vi "Dashboard Main.vi"() -> ()   [LabVIEW 2017]
uses:
  <vilib>/Rock Robotics/WPI/DriverStation/WPI_DriverStationAllianceInfo.ctl
  <vilib>/Rock Robotics/WPI/DriverStation/WPI_DriverStationPositionInfo.ctl
  <vilib>/Rock Robotics/SystemInterfaces/NetworkCommunication/NetComm_MatchType.ctl
  <vilib>/Utility/miscctls.llb/LVRowAndColumnTypeDef.ctl
  <vilib>/event_ctls.llb/eventvkey.ctl
  <vilib>/Rock Robotics/Network Tables/NT Read Numeric Array.vi
  <vilib>/Rock Robotics/Network Tables/NT Write Boolean.vi
  <vilib>/Rock Robotics/WPI/Dashboard/WPI_DashboardLogging Global.vi
panel:
  in  "Camera Name":string(combo)="No Camera Selection"
  out "Camera Info":cluster{"Mbps LED":bool, "Mbps":dbl, "fps":dbl} {"fps" format="%#.1g"; "Mbps" format="%#.1g"}
  in  "Camera Settings":T1={"Frame Rate"=30, "Compression"=30, "Size"=1, "DB Camera Config"=FALSE} {"Frame Rate" scale=1.0..30.0; "Compression" scale=100.0..-1.0; "Size" items=["640x480", "320x240", "160x120"]}
  in  "TCP":refnum<k5>
  out "Robot IP":string
  out "Image Message":string="Timeout in Camera Communications"
  in  "Dashboard Tab":T2(tab)
  out "Cube Lift Height":dbl
  in  "Reset Gyro":bool
  in  "Select Auto":string(combo)="Select Autonomous ..."
  out "NT Connection":bool
  out "MotorChart R":cluster{"Numeric":dbl, "Numeric":dbl}(graph)
  out "MotorChart L":cluster{"Numeric":dbl, "Numeric":dbl}(graph)
  out "MotorSliders R":cluster{"MotorSlide1":dbl, "MotorSlide2":dbl} {"MotorSlide2" scale=-1.0..1.0 scale format="%#_2e"; "MotorSlide1" scale=-1.0..1.0 scale format="%#_2e"}
  out "MotorSliders L":cluster{"MotorSlide1":dbl, "MotorSlide2":dbl} {"MotorSlide2" scale=-1.0..1.0 scale format="%#_2e"; "MotorSlide1" scale=-1.0..1.0 scale format="%#_2e"}
  out "Gyro":dbl(knob) scale=0.0..360.0
  out "JS1 Z":dbl(slide) scale=-1.0..1.0 scale format="%#_2e"
  out "JS1 Graph":cluster{"X":dbl, "Y":dbl}[](graph)
  out "JS1 Buttons":T3
  out "JS2 Z":dbl(slide) scale=-1.0..1.0 scale format="%#_2e"
  out "JS2 Graph":cluster{"X":dbl, "Y":dbl}[](graph)
  out "JS2 Buttons":T3
  out "Mode":T4(ring)=enum."Auto Disabled"
  in  "Rec Mode":enum32{"Stop", "Record", "Playback"}(radio)
  in  "Camera Settings Right":T1={"Frame Rate"=30, "Compression"=30, "Size"=1, "DB Camera Config"=FALSE} {"Frame Rate" scale=1.0..30.0; "Compression" scale=100.0..-1.0; "Size" items=["640x480", "320x240", "160x120"]}
  in  "Camera Name Right":string(combo)="No Camera Selection"
  out "Camera Image Right":T5(plugin-control)
  in  "Cube Lift Up Speed":dbl=10.0 min=0.0 max=10.0 step=1.0
  in  "Robot Lift Speed":dbl=10.0 min=0.0 max=10.0 step=1.0
  in  "H-Wheel Motor Controller Selection":string(combo)="Spark"
  in  "Cube Lift Down Speed":dbl=10.0 min=0.0 max=10.0 step=1.0
  in  "Drive Motor Controller Selection":string(combo)="Talon SRX"
  in  "Y-AXIS":dbl=10.0 min=0.0 max=10.0 step=1.0
  in  "X-AXIS":dbl=10.0 min=0.0 max=10.0 step=1.0
  in  "H-Wheel":dbl=10.0 min=0.0 max=10.0 step=1.0
  out "Event Name":string
  out "Replay Number":u16
  out "Match Type":T6
  out "Match Number":u16
  out "Position":T7
  out "Alliance":T8
  in  "Target Distance":dbl
  out "Inches from Wall":dbl
  in  "Slow Speed":dbl(slide)=0.49999999999999994 scale=0.0..1.0
  in  "Test Slider":dbl(slide) scale=0.0..100.0 scale format="%#_3g"
  in  "On/Off":bool caption="Solenoid"
  in  "Test Name":u16(ring) items=["Select the test to run..."]
  in  "Test Tree":string(tree)
  in  "Motor":cluster{"Value":dbl, "Enable":bool} {"Value" scale=-1.0..1.0 scale format="%#_3g"}
  out "Progress":T9 {"Test Progress" scale=0.0..100.0}
  in  "Rev/Fwd":cluster{"Forward":bool, "Reverse":bool}
  in  "Test Ring":u16(ring) items=["Monochrome", "Color"]
  out "Cmd Status":string
  in  "Execute Command":bool
  in  "Command Params":string[][](table)
  in  "Command Selection":i32(listbox)
  in  "CheckList":i32(listbox)
  out "Tree":string(tree)
  out "Camera Image":T5(plugin-control)
  out "Background":bool
  # "HW"
  # "Joysticks"
  # "Drive Motors"
  # "Front"
  # "Right"
  # "Left"
  # "Back"
  # "HW"
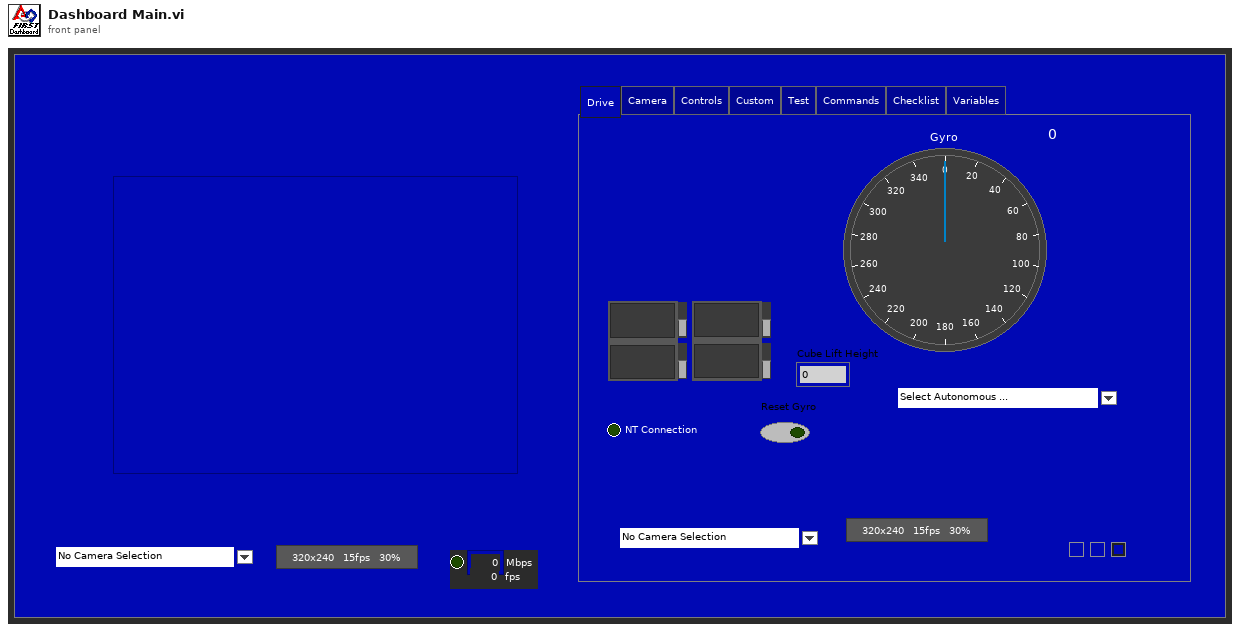
[diagram p1: front panel]
types:
  T1 = cluster{"Frame Rate":i32, "Compression":i32, "Size":u16, "DB Camera Config":bool}
  T2 = enum32{"Drive", "Camera", "Controls", "Custom", "Test", "Commands", "Checklist", "Variables"}
  T3 = cluster{bool, bool, bool, bool, bool, bool, bool, bool, bool, bool, bool, bool}
  T4 = enum8{"Tele-Op Disabled", "Tele-Op Enabled", "Auto Disabled", "Auto Enabled", "Test Disabled", "Test Enabled", "Disconnected", "No Code", "E-Stop"}
  T5 = typedef "IMAQ Image.ctl" = refnum<image>
  T6 = typedef "NetComm_MatchType.ctl" = enum32{"None", "Practice", "Qualification", "Elimination"}
  T7 = typedef "WPI_DriverStationPositionInfo.ctl" = enum16{"1", "2", "3"}
  T8 = typedef "WPI_DriverStationAllianceInfo.ctl" = enum16{"Red", "Blue", "Invalid"}
  T9 = cluster{"Test Progress":u8, "Test Progress Text":string}
  T10 = cluster{"Save Path":path, "Interval (s)":dbl, "Keep":i32}
  T11 = enum32{"Drive", "Camera", "Basic", "Custom", "Test", "Commands", "Checklist", "Variables"}
  T12 = typedef "Image Type" = u32
  T13 = cluster{"IDs":cluster{"RPC field ID":u16, "Unique ID":u16}, "String":string}
  T14 = cluster{"Error Strings":string, "Disable Counts":cluster{u16, u16}, "Rail Faults":cluster{u16, u16, u16}, "Robot IP":string, "DB Mode":u8, "Event Info":cluster{"Name":string, "Type":u8, "Number":u16, "Replay":u8}}
  T15 = cluster{"Storage":cluster{"Disk Free":u64, "RAM Block":u32, "RAM free":u32}, "CPU Utilization":cluster{"CPU % ISR":sgl, "CPU % Time Crit":sgl, "CPU % Timed Str":sgl, "CPU % High":sgl, "CPU % Above":sgl, "CPU % Normal":sgl, "CPU % Low":sgl}, "CAN":cluster{"% Bus Utilization":sgl, "Bus Off Cnt":u32, "TX_FIFO Full Cnt":u32, "Receive Error Cnt":u8, "Transmit Error Cnt":u8}, "HID":cluster{"HID Outputs":u32, "Rumble Low":u16, "Rumble High":u16}[]}
  T16 = cluster{"Status bits":cluster{"Test Mode":bool, "Autonomous":bool, "Enabled":bool, "Code Start":bool, "Brownout":bool, "Reserved 2":bool, "Reserved 3":bool, "E-Stop":bool}, "Code Trace":cluster{"Disabled":bool, "TeleOp":bool, "Auto":bool, "Test":bool}, "Controller Type":enum16{"unknown", "cRIO", "roboRio"}, "Code?":enum16{"unknown", "noCode", "code"}, "Battery V":dbl}
  T17 = cluster{"Control Bits":cluster{"TestMode":bool, "Autonomous":bool, "Enabled":bool, "FMS Present":bool, bool, bool, bool, "E-Stop":bool}, "Team Station ":u8, "Countdown":sgl, "Joystick Values":cluster{"Axes":dbl[], "Buttons":bool[], "POVs":i16[]}[]}
  T18 = cluster{"Axes":dbl[], "Buttons":bool[], "POVs":i16[]}[]
  T19 = cluster{"Axes":dbl[], "Buttons":bool[], "POVs":i16[]}
  T20 = cluster{"Buttons[0]":bool, "Buttons[1]":bool, "Buttons[2]":bool, "Buttons[3]":bool, "Buttons[4]":bool, "Buttons[5]":bool, "Buttons[6]":bool, "Buttons[7]":bool, "Buttons[8]":bool, "Buttons[9]":bool, "Buttons[10]":bool, "Buttons[11]":bool}
  T21 = cluster{"Camera Image":refnum<vi>, "Dashboard Tab":refnum<vi>, "Background":refnum<vi>, "Rec Mode":refnum<vi>, "Test Slider":refnum<vi>, "On/Off ":refnum<vi>, "Test Ring":refnum<vi>, "Rev/Fwd":refnum<vi>, "Test Name":refnum<vi>, "Motor":refnum<vi>, "Progress":refnum<vi>, "CheckList":refnum<vi>, "Tree":refnum<vi>, "Test Tree":refnum<vi>, "Command Params":refnum<vi>, "Command Selection":refnum<vi>, "Execute Command":refnum<vi>, "Cmd Status":refnum<vi>, "Camera Settings":refnum<vi>, "Camera Name":refnum<vi>, "Camera Info":refnum<vi>, "Camera Settings Right":refnum<vi>, "Camera Name Right":refnum<vi>, "Camera Image Right":refnum<vi>}
  T22 = cluster{"Camera Name":string, string, "Saved DB Images Info":cluster{"Save Path":path, "Interval (s)":dbl, "Keep":i32}}
  T23 = cluster{"Camera Name Right":string, string, "Saved DB Images Info":cluster{"Save Path":path, "Interval (s)":dbl, "Keep":i32}}
  T24 = cluster{"Operation":enum16{"Update", "Clear"}, "Color Box":u32}[]
  T25 = typedef "eventvkey.ctl" = enum16{"ASCII", "Enter", "Return", "Shift", "Ctrl", "Alt", "Cmd", "Opt", "Caps", "NumLock", "Clear", "Break", "Up", "Down", "Left", "Right", "Insert", "Delete", "Home", "End", "PageUp", "PageDown", "Escape", "Help", "Pause", "ScrollLock", "F1", "F2", "F3", "F4", "F5", "F6", "F7", "F8", "F9", "F10", "F11", "F12", "F13", "F14", "F15", "F16", "F17", "F18", "F19", "F20", "F21", "F22", "F23", "F24", "Play", "VolumeUp", "VolumeDown", "Mute", "Two Byte Char"}
  T26 = cluster{"Image Size":bool, "Image Type":bool, "Pixel Value":bool, "ROI Information":bool, "Zoom Factor":bool}
  T27 = cluster{"Operation":enum16{"Update", "Clear"}, "Color Box":u32}
  T28 = typedef "LVRowAndColumnTypeDef.ctl" = cluster{"Row":i32, "Column":i32}
  T29 = cluster{"Shift":bool, "Ctrl":bool, "Alt":bool, "Cmd":bool, "Opt":bool}
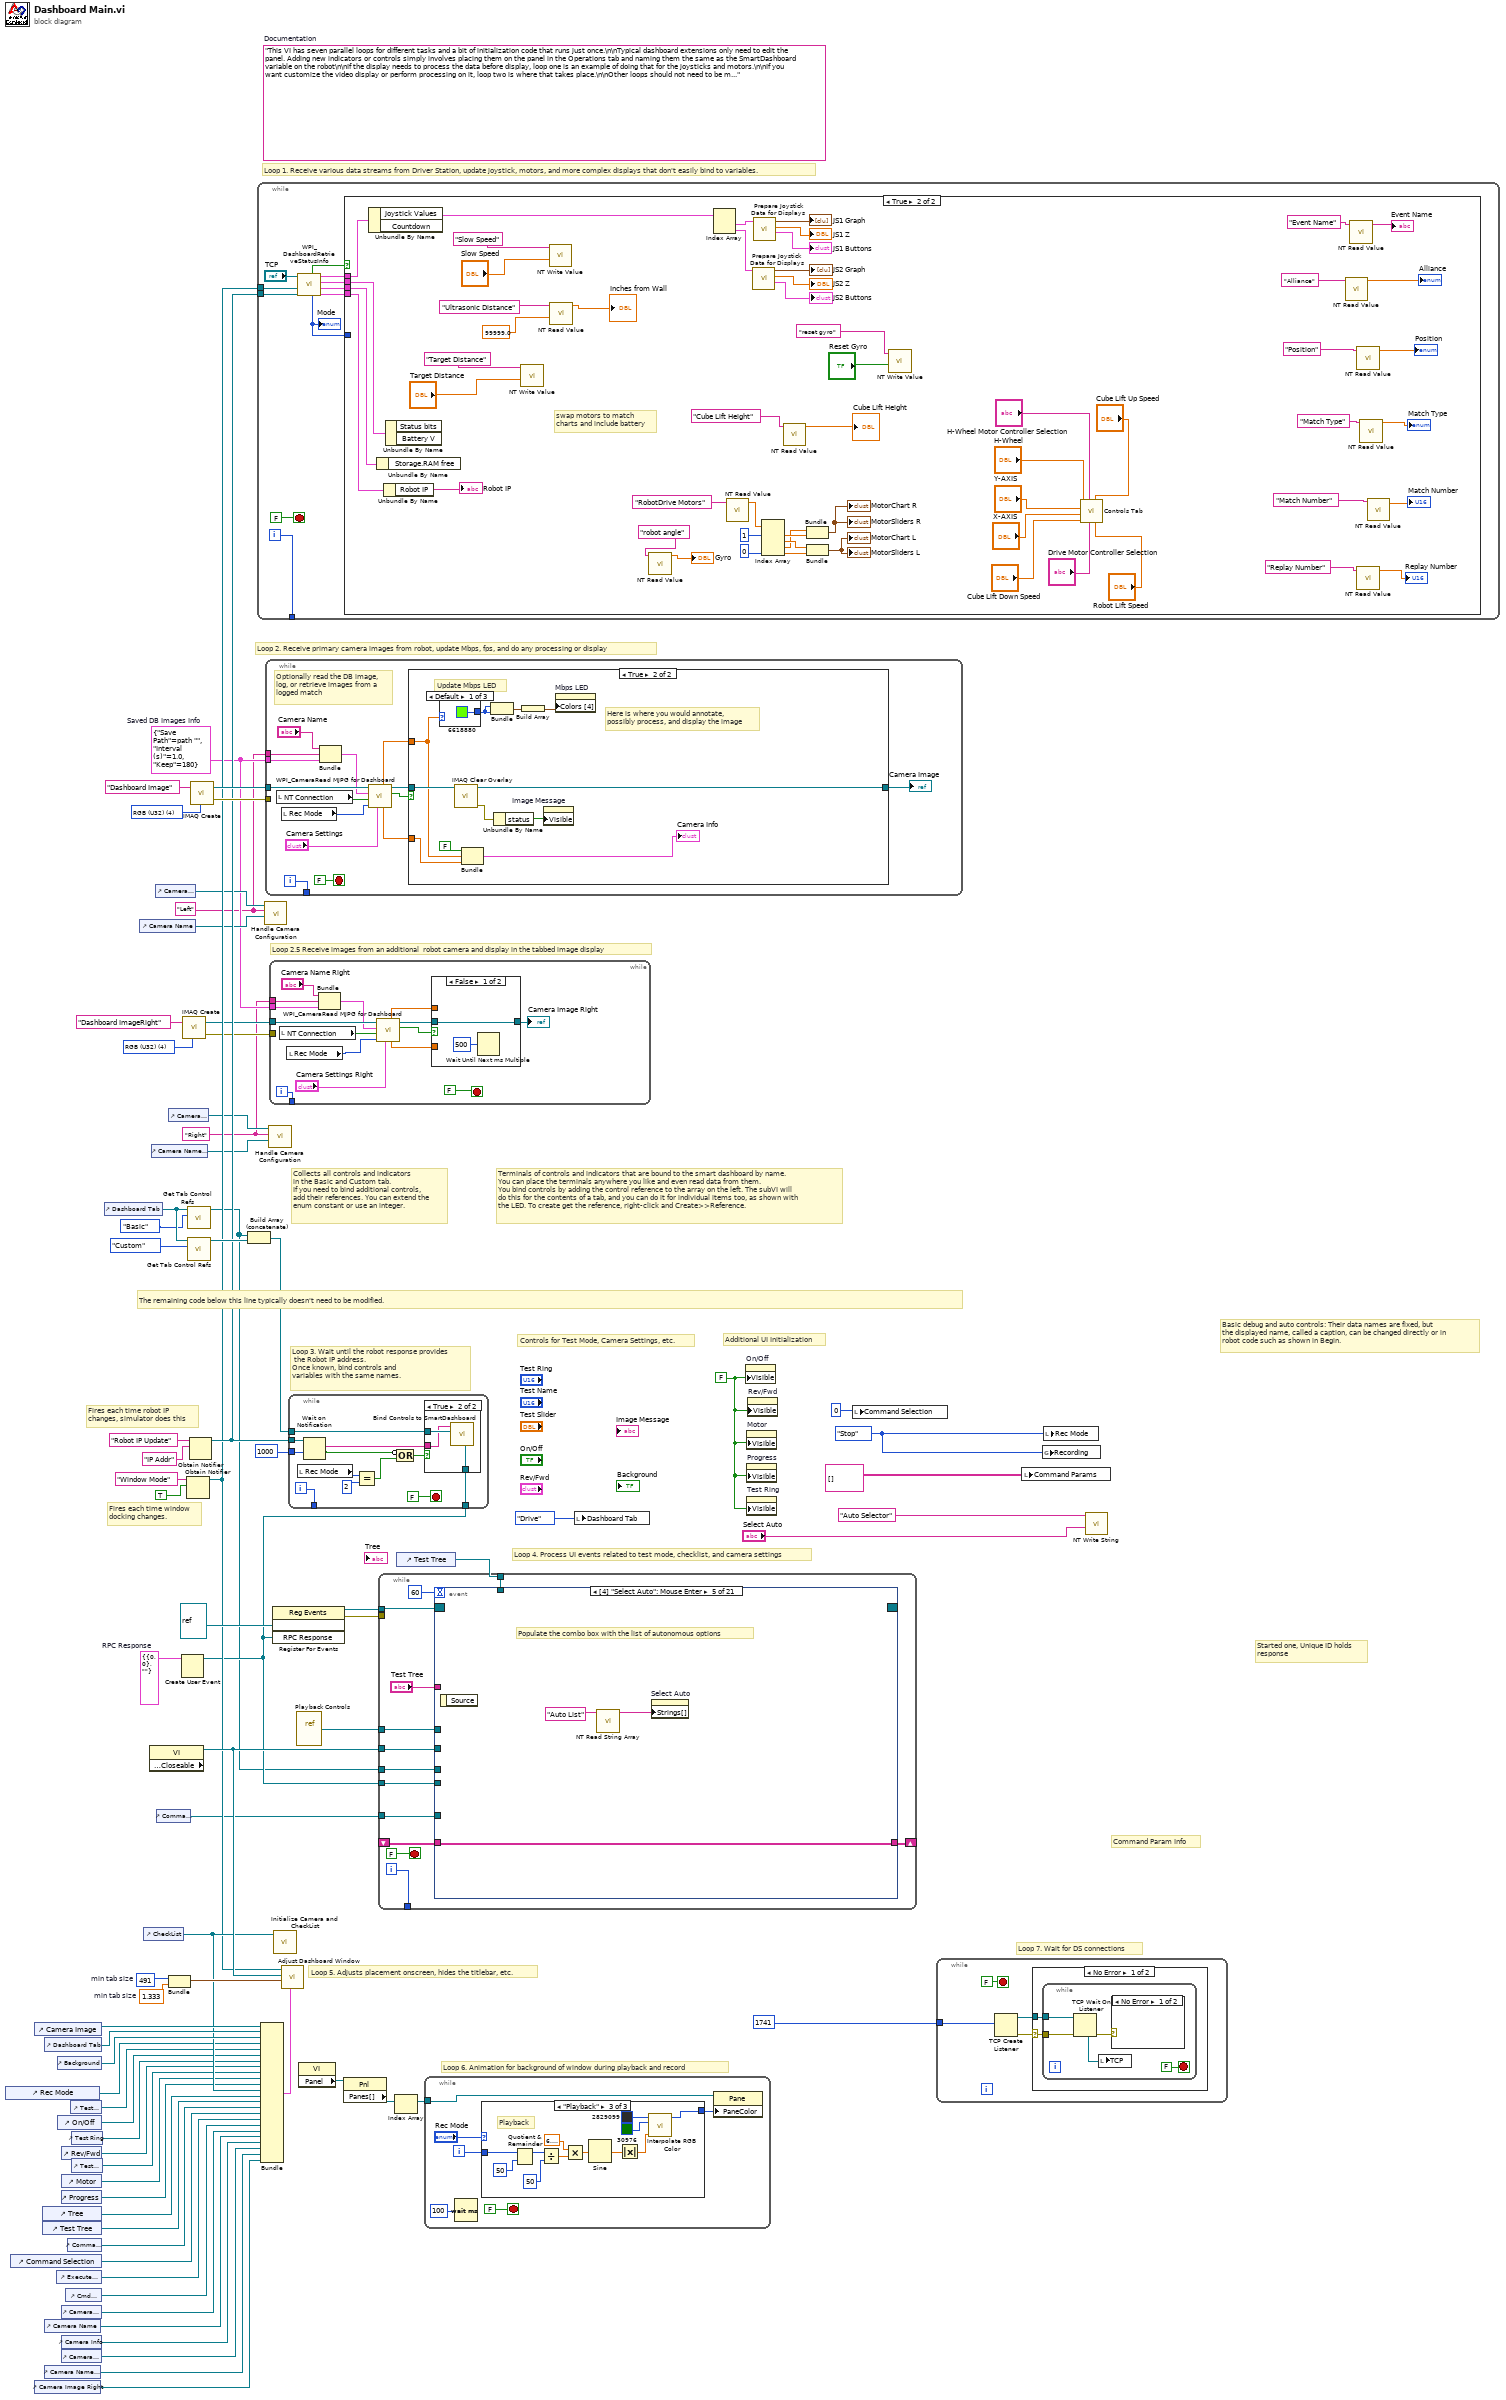
[diagram p0: block diagram]
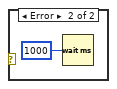
[diagram p3: hidden frame]
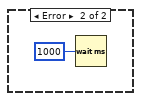
[diagram p4: hidden frame]
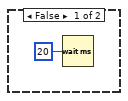
[diagram p5: hidden frame]
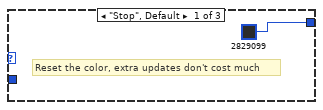
[diagram p6: hidden frame]
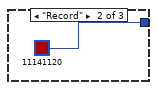
[diagram p7: hidden frame]
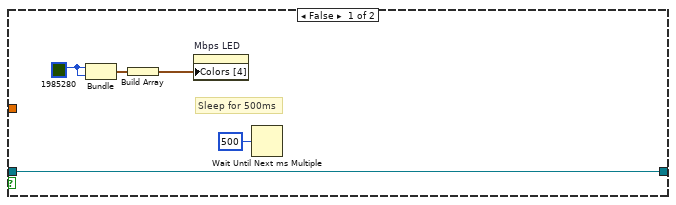
[diagram p9: hidden frame]
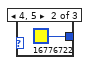
[diagram p10: hidden frame]
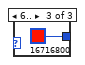
[diagram p11: hidden frame]
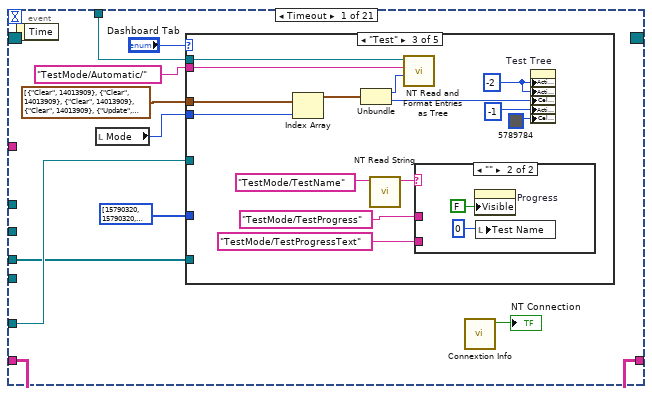
[diagram p12: hidden frame]
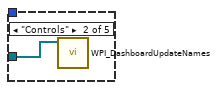
[diagram p14: hidden frame]
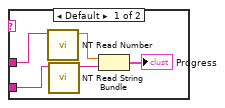
[diagram p15: hidden frame]
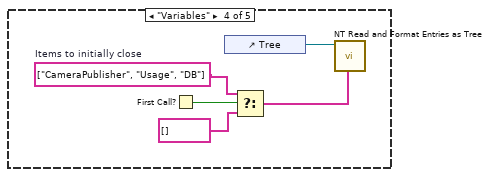
[diagram p16: hidden frame]
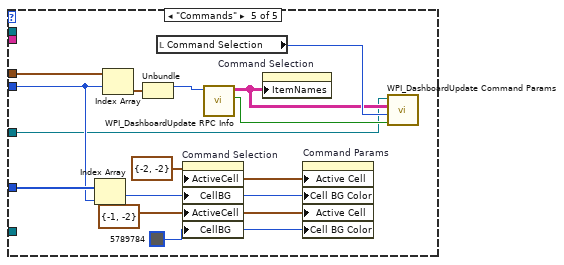
[diagram p17: hidden frame]
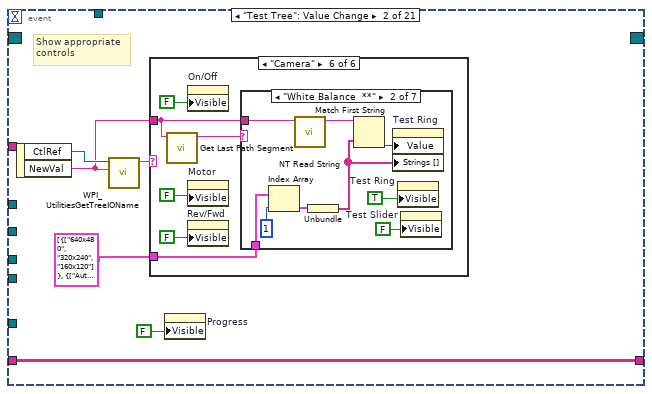
[diagram p18: hidden frame]
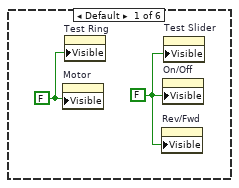
[diagram p19: hidden frame]
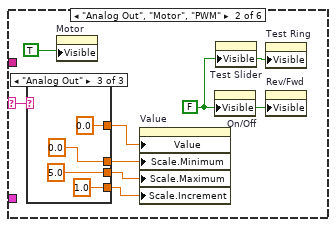
[diagram p20: hidden frame]
diagram:
  w3 = T10 {"Save Path"=path "", "Interval (s)"=1.0, "Keep"=180}  # Saved DB Images Info
  w2 = "Right"
  w1 = "Left"
  w13 = T12 4 items=["Grayscale (U8)", "Grayscale (I16)", "Grayscale (SGL)", "Complex (CSG)", "RGB (U32)", "HSL (U32)", "RGB (U64)"] ("Image Type")
  w29 = T13 {"IDs"={"RPC field ID"=0, "Unique ID"=0}, "String"=""}  # RPC Response
  w52 = 491  # min tab size
  w51 = 1.333  # min tab size
  w59 = enum32{"Stop", "Record", "Playback"}."Stop" ("Rec Mode")
  w36 = FALSE ("Visible")
  (unwired) "This VI has seven parallel loops for different tasks and a bit of initialization code that runs just once.\n\nTypical dashboard extensions only need to edit the panel. Adding new indicators or controls simply involves placing them on the panel in the Operations tab and naming them the same as the SmartDashboard variable on the robot\n\nIf the display needs to process the data before display, loop one is an example of doing that for the joysticks and motors.\n\nIf you want customize the video display or perform processing on it, loop two is where that takes place.\n\nOther loops should not need to be modified. They are pretty standard, and document the task they perform."  # Documentation
  w76 = T12 4 items=["Grayscale (U8)", "Grayscale (I16)", "Grayscale (SGL)", "Complex (CSG)", "RGB (U32)", "HSL (U32)", "RGB (U64)"] ("Image Type")
  # "Loop 2.5 Receive images from an additional  robot camera and display in the tabbed image display"
  # "Command Param Info"
  # "Started one, Unique ID holds\nresponse"
  # "Loop 7. Wait for DS connections"
  # "Basic debug and auto controls: Their data names are fixed, but\nthe displayed name, called a caption, can be changed directly or in\nrobot code such as shown in Begin."
  # "Controls for Test Mode, Camera Settings, etc."
  # "Additional UI Initialization"
  # "Loop 6. Animation for background of window during playback and record"
  # "Fires each time robot IP\nchanges, simulator does this"
  # "Fires each time window\ndocking changes."
  # "Collects all controls and indicators\nin the Basic and Custom tab.\nIf you need to bind additional controls,\nadd their references. You can extend the\nenum constant or use an integer."
  # "The remaining code below this line typically doesn't need to be modified."
  # "Loop 4. Process UI events related to test mode, checklist, and camera settings"
  # "Terminals of controls and indicators that are bound to the smart dashboard by name.\nYou can place the terminals anywhere you like and even read data from them.\nYou bind controls by adding the control reference to the array on the left. The subVI will\ndo this for the contents of a tab, and you can do it for individual items too, as shown with\nthe LED. To create get the reference, right-click and Create>>Reference."
  # "Loop 3. Wait until the robot response provides\n the Robot IP address.\nOnce known, bind controls and\nvariables with the same names."
  # "Loop 5. Adjusts placement onscreen, hides the titlebar, etc."
  # "Loop 1. Receive various data streams from Driver Station, update joystick, motors, and more complex displays that don't easily bind to variables."
  # "Loop 2. Receive primary camera images from robot, update Mbps, fps, and do any processing or display"
  n1 = control-ref of="Rec Mode"() -> (w42:refnum<vi>)
  n2 = control-ref of="Command Selection"() -> (w28:refnum<vi>)
  n3 = control-ref of="Camera Image Right"() -> (w6:refnum<vi>)
  n4 = control-ref of="Camera Image"() -> (w54:refnum<vi>)
  n5 = control-ref of="Tree"() -> (w46:refnum<vi>)
  n6 = control-ref of="Test Tree"() -> (w45:refnum<vi>)
  n7 = control-ref of="Dashboard Tab"() -> (w53:refnum<vi>)
  n8 = control-ref of="Camera Name"() -> (w19:refnum<vi>)
  n9 = control-ref of="Camera Name Right"() -> (w7:refnum<vi>)
  n10 = control-ref of="Execute Command"() -> (w30:refnum<vi>)
  n11 = control-ref of="Background"() -> (w49:refnum<vi>)
  n12 = control-ref of="On/Off"() -> (w40:refnum<vi>)
  n13 = control-ref of="Progress"() -> (w37:refnum<vi>)
  n14 = control-ref of="Camera Settings"() -> (w20:refnum<vi>)
  n15 = control-ref of="Camera Info"() -> (w18:refnum<vi>)
  n16 = control-ref of="Camera Settings Right"() -> (w8:refnum<vi>)
  n17 = control-ref of="Rev/Fwd"() -> (w38:refnum<vi>)
  n18 = control-ref of="Motor"() -> (w43:refnum<vi>)
  n19 = control-ref of="Cmd Status"() -> (w24:refnum<vi>)
  n20 = control-ref of="Command Params"() -> (w31:refnum<vi>)
  n21 = control-ref of="Test Slider"() -> (w41:refnum<vi>)
  n22 = control-ref of="Test Ring"() -> (w39:refnum<vi>)
  n23 = control-ref of="Test Name"() -> (w44:refnum<vi>)
  n24 = control-ref of="Dashboard Tab"() -> (w57:refnum<vi>)
  n25 = control-ref of="Camera Name"() -> (w21:refnum<vi>)
  n26 = control-ref of="CheckList"() -> (w47:refnum<vi>)
  n27 = property class="VI" props=["Front Panel.Closeable"]() -> (reference out=w58:refnum<vi>)  [unwired: 2 in, 2 out]
  n28 = control-ref of="Camera Name Right"() -> (w9:refnum<vi>)
  n29 = control-ref of="Camera Settings"() -> (w22:refnum<vi>)
  n30 = control-ref of="Command Params"() -> (w23:refnum<vi>)
  n31 = control-ref of="Camera Settings Right"() -> (w10:refnum<vi>)
  n32 = Bundle("min tab size"=w52, "min tab size"=w51) -> (w50:cluster{"min tab size":i32, "min tab size":dbl})  [unwired: 1 in]
  n33 = Create User Event(user event datatype=w29) -> (user event=w25:refnum<user-event>)  [unwired: 1 in, 1 out]
  n34 = call "IMAQ Create"("Image Name"="Dashboard ImageRight", "Image Type"=w13) -> ("New Image"=w12:T5, "error out"=w11:errorcluster)  [unwired: 2 in, 1 out]
  n35 = Obtain Notifier(name (unnamed)="Window Mode", notification data type=TRUE) -> (notifier out=w34:refnum<notifier>)  [unwired: 2 in, 2 out]
  n36 = call <vilib>:"Get Tab Control Refs.vi"("Page Index"=T11."Basic" ("Dashboard Tab"), "TabControl in"=w57) -> ("ControlsOnPage"=w17:refnum<vi>[])  [unwired: 9 in]
  n37 = call <vilib>:"Get Tab Control Refs.vi"("Page Index"=T11."Custom" ("Dashboard Tab"), "TabControl in"=w57) -> ("ControlsOnPage"=w56:refnum<vi>[])  [unwired: 9 in]
  n38 = Obtain Notifier(name (unnamed)="Robot IP Update", notification data type="IP Addr" ("name (unnamed)")) -> (notifier out=w35:refnum<notifier>)  [unwired: 2 in, 2 out]
  n39 = call "IMAQ Create"("Image Name"="Dashboard Image", "Image Type"=w76) -> ("New Image"=w74:T5, "error out"=w73:errorcluster)  [unwired: 2 in, 1 out]
  n40 = Build Array (concatenate)(w17, w56) -> (w55:refnum<vi>[])
  n41 = while {
    tunnel: [w86] -> _
    tunnel: w35 -> [w80]
    tunnel: w34 -> [w77]
    i -> [w86]
    stop <- FALSE stop-if-true
    n42 = call <vilib>:"WPI_DashboardRetrieveStatusInfo.vi"("Binding Refnum"=w80, "Window Mode Notifier"=w77, "TCP Cnx"="TCP") -> ("Power and Errors"=w81:T14, "Robot Metrics"=w84:T15, "Status Info"=w85:T16, "Control Info"=w82:T17, "Robot Mode"=w79:T4, "Process?"=w83:bool)  [unwired: 3 in]
    "Mode" <- w79
    n43 = case shown="True" w83 {
      tunnel: w85 -> [_ w145]
      tunnel: w84 -> [_ w144]
      tunnel: w82 -> [_ w143]
      tunnel: w81 -> [_ w142]
      tunnel: w79 -> [_ _]
      frame False {
        n44 = Wait (ms)(milliseconds to wait=u32 20) -> ()  [unwired: 1 out]
      }
      frame True {
        # "swap motors to match\ncharts and include battery"
        n45 = Unbundle By Name(w143) -> ("Joystick Values"=w133:T18)  [unwired: 1 out]
        n46 = Unbundle By Name(w144) -> ()  [unwired: 1 out]
        n47 = Unbundle By Name(w142) -> ("Robot IP"=→"Robot IP":string)
        n48 = Unbundle By Name(w145) -> ()  [unwired: 2 out]
        n49 = call-poly <vilib>:"NT Write Value.vi"("Numeric"="Target Distance", "Name"="Target Distance") -> ()  [unwired: 9 in, 1 out]
        n50 = call-poly <vilib>:"NT Write Value.vi"("Numeric"="Slow Speed", "Name"="Slow Speed") -> ()  [unwired: 9 in, 1 out]
        n51 = call-poly <vilib>:"NT Read Value.vi"("Default Value"=99999.0, "Name"="Ultrasonic Distance") -> ("Numeric"=→"Inches from Wall":dbl)  [unwired: 8 in, 1 out]
        n52 = call-poly <vilib>:"NT Read Value.vi"("Name"="robot angle") -> ("Numeric"=→"Gyro":dbl)  [unwired: 9 in, 1 out]
        n53 = Index Array(array=w133) -> (element #1=w132:T19, element #2=w128:T19)  [unwired: 2 in]
        n54 = call-poly <vilib>:"NT Read Value.vi"("Name"="RobotDrive Motors") -> ("Numeric Array"=w123:dbl[])  [unwired: 9 in, 1 out]
        n55 = call "Prepare Joystick Data for Displays.vi"("Joystick Values"=w128) -> ("Buttons"=→"JS2 Buttons":T20, "Z Axis"=→"JS2 Z":dbl, "Cartesian Data"=→"JS2 Graph":cluster{"X axis":dbl, "X axis":dbl}[])  [unwired: 8 in]
        n56 = call "Prepare Joystick Data for Displays.vi"("Joystick Values"=w132) -> ("Buttons"=→"JS1 Buttons":T20, "Z Axis"=→"JS1 Z":dbl, "Cartesian Data"=→"JS1 Graph":cluster{"X axis":dbl, "X axis":dbl}[])  [unwired: 8 in]
        n57 = Index Array(array=w123, index #1=1, index #4=0) -> (element #1=w137:dbl, element #2=w138:dbl, element #3=w136:dbl, element #4=w141:dbl)  [unwired: 2 in]
        n58 = call-poly <vilib>:"NT Read Value.vi"("Name"="Cube Lift Height") -> ("Numeric"=→"Cube Lift Height":dbl)  [unwired: 9 in, 1 out]
        n59 = Bundle("Numeric"=w136, "Numeric"=w137) -> (→"MotorChart R" →"MotorSliders R":cluster{"Numeric":dbl, "Numeric":dbl})  [unwired: 1 in]
        n60 = Bundle("Numeric"=w138, "Numeric"=w141) -> (→"MotorChart L" →"MotorSliders L":cluster{"Numeric":dbl, "Numeric":dbl})  [unwired: 1 in]
        n61 = call-poly <vilib>:"NT Write Value.vi"("Boolean"="Reset Gyro", "Name"="reset gyro") -> ()  [unwired: 9 in, 1 out]
        n62 = call "Controls Tab.vi"("Robot Lift Motor"="Robot Lift Speed", "Cube Lift Up Motor"="Cube Lift Up Speed", "Motor Controller Selection"="Drive Motor Controller Selection", "H-Wheel Motor Controller Selection"="H-Wheel Motor Controller Selection", "Cube Lift Down Motor"="Cube Lift Down Speed", "X-AXIS"="X-AXIS", "Y-AXIS"="Y-AXIS", "H-Wheel"="H-Wheel") -> ()  [unwired: 4 in]
        n63 = call-poly <vilib>:"NT Read Value.vi"("Name"="Alliance") -> ("Numeric"=→"Alliance":dbl)  [unwired: 9 in, 1 out]
        n64 = call-poly <vilib>:"NT Read Value.vi"("Name"="Event Name") -> ("String"=→"Event Name":string)  [unwired: 9 in, 1 out]
        n65 = call-poly <vilib>:"NT Read Value.vi"("Name"="Position") -> ("Numeric"=→"Position":dbl)  [unwired: 9 in, 1 out]
        n66 = call-poly <vilib>:"NT Read Value.vi"("Name"="Replay Number") -> ("Numeric"=→"Replay Number":dbl)  [unwired: 9 in, 1 out]
        n67 = call-poly <vilib>:"NT Read Value.vi"("Name"="Match Type") -> ("Numeric"=→"Match Type":dbl)  [unwired: 9 in, 1 out]
        n68 = call-poly <vilib>:"NT Read Value.vi"("Name"="Match Number") -> ("Numeric"=→"Match Number":dbl)  [unwired: 9 in, 1 out]
      }
    }
  }
  n69 = Bundle("Camera Image"=w54, "Dashboard Tab"=w53, "Background"=w49, "Rec Mode"=w42, "Test Slider"=w41, "On/Off"=w40, "Test Ring"=w39, "Rev/Fwd"=w38, "Test Name"=w44, "Motor"=w43, "Progress"=w37, "CheckList"=w47, "Tree"=w46, "Test Tree"=w45, "Command Params"=w31, "Command Selection"=w28, "Execute Command"=w30, "Cmd Status"=w24, "Camera Settings"=w20, "Camera Name"=w19, "Camera Info"=w18, "Camera Settings Right"=w8, "Camera Name Right"=w7, "Camera Image Right"=w6) -> (w48:T21)  [unwired: 1 in]
  n70 = call "Handle Camera Configuration.vi"("CameraNameRef"=w21, "Display Name"=w1, "ClusterRef"=w22) -> ()  [unwired: 9 in]
  n71 = while {
    tunnel: w74 -> [w158]
    tunnel: w73 -> [_]
    tunnel: [w159] -> _
    tunnel: w3 -> [w149]
    tunnel: w1 -> [w146]
    i -> [w159]
    stop <- FALSE stop-if-true
    # "Optionally read the DB image,\nlog, or retrieve images from a\nlogged match"
    n72 = local read "NT Connection"() -> (w150:bool)
    n73 = local read "Rec Mode"() -> (w154:enum32{"Stop", "Record", "Playback"})
    n74 = Bundle("Camera Name"="Camera Name", w146, "Saved DB Images Info"=w149) -> (w148:T22)  [unwired: 1 in]
    n75 = call <vilib>:"WPI_CameraRead MJPG for Dashboard.vi"("Camera Settings"="Camera Settings", "Rec Mode"=w154, "NT Connection"=w150, "Capture Info"=w148, "Refnum in"=w158) -> ("Active"=w156:bool, "Refnum out"=w157:T5, "FPS"=w155:dbl, "Bandwidth (Mbps)"=w153:dbl)  [unwired: 3 in]
    n76 = case shown="True" w156 {
      tunnel: w157 -> [w161 w172]
      tunnel: w153 -> [_ w169]
      tunnel: w155 -> [_ w170]
      tunnel: [w161 w166] -> w151
      frame False {
        w163 = u32 1985280 ("Color Box")
        # "Sleep for 500ms"
        n77 = Bundle("Color Box"=w163, "Color Box"=w163) -> (w164:cluster{"Color Box":u32, "Color Box":u32})  [unwired: 1 out]
        n78 = Build Array(w164) -> (w162:cluster{"Color Box":u32, "Color Box":u32}[])
        n79 = property on="Mbps LED" class="Bool (strict)"("Colors [4]"=w162) -> ()  [unwired: 2 in, 2 out]
        n80 = Wait Until Next ms Multiple(millisecond multiple=u32 500) -> ()  [unwired: 1 out]
      }
      frame True {
        # "Here is where you would annotate,\npossibly process, and display the image"
        # "Update Mbps LED"
        n81 = case shown="Default" w169 {
          tunnel: [u32 6618880 ("Color Box") u32 16776722 ("Color Box") u32 16716800 ("Color Box")] -> w173
          frame Default {
          }
          frame 4, 5 {
          }
          frame 6.. {
          }
        }
        n82 = call "IMAQ Clear Overlay"("Image"=w172) -> ("error out"=w175:errorcluster, "Image Out"=w166:T5)  [unwired: 2 in, 7 out]
        n83 = Bundle(FALSE, "Bandwidth (Mbps)"=w169, "FPS"=w170) -> (→"Camera Info":cluster{bool, "Bandwidth (Mbps)":dbl, "FPS":dbl})  [unwired: 1 in]
        n84 = Bundle("Color Box"=w173, "Color Box"=w173) -> (w174:cluster{"Color Box":u32, "Color Box":u32})  [unwired: 1 out]
        n85 = Unbundle By Name(w175) -> ("status"=w176:bool)
        n86 = Build Array(w174) -> (w171:cluster{"Color Box":u32, "Color Box":u32}[])
        n87 = property on="Image Message" class="Str"("Visible"=w176) -> ()  [unwired: 2 in, 2 out]
        n88 = property on="Mbps LED" class="Bool (strict)"("Colors [4]"=w171) -> ()  [unwired: 2 in, 2 out]
      }
    }
    "Camera Image" <- w151
  }
  n89 = call "Handle Camera Configuration.vi"("CameraNameRef"=w9, "Display Name"=w2, "ClusterRef"=w10) -> ()  [unwired: 9 in]
  n90 = while {
    tunnel: w12 -> [w194]
    tunnel: w11 -> [_]
    tunnel: [w189] -> _
    tunnel: w3 -> [w183]
    tunnel: w2 -> [w180]
    i -> [w189]
    stop <- FALSE stop-if-true
    n91 = local read "NT Connection"() -> (w184:bool)
    n92 = local read "Rec Mode"() -> (w193:enum32{"Stop", "Record", "Playback"})
    n93 = Bundle("Camera Name Right"="Camera Name Right", w180, "Saved DB Images Info"=w183) -> (w182:T23)  [unwired: 1 in]
    n94 = call <vilib>:"WPI_CameraRead MJPG for Dashboard.vi"("Camera Settings"="Camera Settings Right", "Rec Mode"=w193, "NT Connection"=w184, "Capture Info"=w182, "Refnum in"=w194) -> ("Active"=w188:bool, "Refnum out"=w191:T5, "FPS"=w186:dbl, "Bandwidth (Mbps)"=w187:dbl)  [unwired: 3 in]
    n95 = case shown="False" w188 {
      tunnel: w191 -> [w195 w197]
      tunnel: w187 -> [_ _]
      tunnel: w186 -> [_ _]
      tunnel: [w195 w197] -> w185
      frame False {
        n96 = Wait Until Next ms Multiple(millisecond multiple=u32 500) -> ()  [unwired: 1 out]
      }
      frame True {
      }
    }
    "Camera Image Right" <- w185
  }
  n97 = register-events(refnum<vi> refnum, w25) -> (reference out=w63:refnum<event-registration>, error out=w62:errorcluster)  [unwired: 2 in]
  n98 = call "Initialize Camera and CheckList.vi"("ListBox in"=w47) -> ()  [unwired: 11 in]
  n99 = call "Adjust Dashboard Window.vi"("Sizing Refnums"=w48, "Size Constraints"=w50, "VI"=w58, "WIn Mode"=w34) -> ()  [unwired: 8 in]
  n100 = while {
    tunnel: w55 -> [w209]
    tunnel: w35 -> [w207]
    tunnel: [w205] -> _
    tunnel: u32 1000 ("milliseconds to wait") -> [w204]
    tunnel: w25 -> [w198]
    i -> [w205]
    stop <- FALSE stop-if-true
    n101 = local read "Rec Mode"() -> (w200:enum32{"Stop", "Record", "Playback"})
    n102 = Wait on Notification(notifier=w207, timeout in ms (-1)=w204) -> (notification=w206:string, timed out?=w202:bool)  [unwired: 2 in, 2 out]
    n103 = Equal?(x=w200, y=u16 2 ("Rec Mode")) -> (x = y?=w201:bool)
    n104 = Compound Arithmetic op=OR(invert w202, w201) -> (w203:bool)
    n105 = case shown="True" w203 {
      tunnel: w209 -> [_ w212]
      tunnel: w206 -> [_ w211]
      tunnel: w198 -> [_ w210]
      frame False {
      }
      frame True {
        n106 = call <vilib>:"Bind Controls to SmartDashboard.vi"("RPC ref"=w210, "Bound Control Refs"=w212, "Server IP Address"=w211) -> ()  [unwired: 9 in]
      }
    }
  }
  n107 = vi-ref "Playback Controls.vi"() -> (w64:refnum<vi>)
  n108 = property class="VI"() -> ("Panel"=w66:refnum<vi>)  [unwired: 2 in, 2 out]
  n109 = property class="Pnl"(reference=w66) -> ("Panes[]"=w67:refnum<vi>[])  [unwired: 1 in, 2 out]
  n110 = Index Array(array=w67) -> (element=w65:refnum<vi>)  [unwired: 1 in]
  n111 = control-ref of="Test Tree"() -> (w68:refnum<vi>)
  n112 = while {
    tunnel: [w222] -> _
    tunnel: w68 -> [w221]
    tunnel: w64 -> [w220]
    tunnel: w63 -> [w219]
    tunnel: w62 -> [_]
    tunnel: w58 -> [w218]
    tunnel: w25 -> [w217]
    tunnel: w23 -> [w216]
    shift-right: [w215] -> _
    shift-left: _ -> [w214]
    tunnel: w17 -> [w213]
    i -> [w222]
    stop <- FALSE stop-if-true
    n113 = event shown="[4] \"Select Auto\": Mouse Enter" {
      selector: w219 -> [_ _ _ _ _ _ _ _ _ _ _ _ _ _ _ _ _ _ _ _ _]
      dyn-events: [_ _ _ _ _ _ _ _ _ _ _ _ _ _ _ _ w482 _ _ _ _] -> _
      timeout: u32 60 ("milliseconds to wait") -> [_ _ _ _ _ _ _ _ _ _ _ _ _ _ _ _ _ _ _ _ _]
      tunnel: w221 -> [w234 _ _ _ _ _ _ _ _ _ _ _ _ _ _ _ _ _ _ _ _]
      tunnel: "Test Tree" -> [_ _ _ _ _ _ _ _ _ _ _ w449 w457 w459 w463 w471 _ _ _ _ _]
      tunnel: w220 -> [_ _ _ _ _ _ _ _ _ _ _ _ _ _ _ _ w484 _ w502 _ _]
      tunnel: w218 -> [_ _ _ _ _ _ _ _ _ _ _ _ _ _ _ _ w480 _ _ _ _]
      tunnel: w217 -> [_ _ _ _ _ _ _ _ _ _ _ _ _ _ _ _ w478 _ _ _ _]
      tunnel: w216 -> [w229 _ _ _ _ _ w400 _ _ _ _ _ _ _ _ _ _ _ _ _ _]
      tunnel: [w228 w277 w379 w384 w393 w397 w398 w407 w417 w424 w436 w448 w455 w458 w462 w470 w477 w497 w499 w503 w516] -> w215
      tunnel: w214 -> [w228 w277 w379 w384 w393 w397 w398 _ _ w424 w436 w448 w455 w458 w462 w470 w477 w497 w499 w503 w516]
      tunnel: w213 -> [w226 _ _ _ _ _ _ _ _ _ _ _ _ _ _ _ _ _ _ _ _]
      event Timeout {
        n114 = event-data() -> ()  [unwired: 1 in, 1 out]
        n115 = local read "Mode"() -> (w231:T4)
        n116 = case shown="\"Test\"" "Dashboard Tab" {
          tunnel: w234 -> [_ _ w250 _ _]
          tunnel: "TestMode/Automatic/" ("Name Pattern") -> [_ _ w249 _ _]
          tunnel: T24 [{"Operation"=enum."Clear", "Color Box"=14013909}, {"Operation"=enum."Clear", "Color Box"=14013909}, {"Operation"=enum."Clear", "Color Box"=14013909}, {"Operation"=enum."Clear", "Color Box"=14013909}, {"Operation"=enum."Update", "Color Box"=14013909}, {"Operation"=enum."Update", "Color Box"=16777215}, {"Operation"=enum."Clear", "Color Box"=14013909}, {"Operation"=enum."Clear", "Color Box"=14013909}, {"Operation"=enum."Clear", "Color Box"=14013909}] -> [_ _ w242 _ w270]
          tunnel: w231 -> [_ _ w241 _ w269]
          tunnel: u32[] [15790320, 15790320, 15790320, 15790320, 16777215, 16777215, 15790320, 15790320, 15790320] -> [_ _ _ _ w275]
          tunnel: w229 -> [_ _ _ _ w263]
          tunnel: w226 -> [_ w236 _ _ _]
          frame "Custom", Default {
          }
          frame "Controls" {
            n117 = call <vilib>:"WPI_DashboardUpdateNames.vi"("Controls on Tab"=w236) -> ()  [unwired: 11 in]
          }
          frame "Test" {
            w248 = -2 ("Active Item:Row Number")
            n118 = Index Array(array=w242, index=w241) -> (element=w243:T27)
            n119 = Unbundle(w243) -> ("Operation"=w244:enum16{"Update", "Clear"}, "Color Box"=w245:u32)
            n120 = call <vilib>:"NT Read String.vi"("Name"="TestMode/TestName") -> ("String"=w239:string)  [unwired: 9 in, 1 out]
            n121 = call <vilib>:"NT Read and Format Entries as Tree.vi"("Operation"=w244, "Name Pattern"=w249, "Tree Refnum"=w250) -> ()  [unwired: 7 in, 2 out]
            n122 = case shown="\"\"" w239 {
              tunnel: "TestMode/TestProgress" ("Name") -> [w252 _]
              tunnel: "TestMode/TestProgressText" ("Name") -> [w251 _]
              frame Default {
                n123 = call <vilib>:"NT Read Number.vi"("Name"=w252) -> ("Numeric"=w253:dbl)  [unwired: 9 in, 1 out]
                n124 = call <vilib>:"NT Read String.vi"("Name"=w251) -> ("String"=w254:string)  [unwired: 9 in, 1 out]
                n125 = Bundle("Numeric"=w253, "String"=w254) -> (→"Progress":cluster{"Numeric":dbl, "String":string})  [unwired: 1 in]
              }
              frame "" {
                n126 = property on="Progress" class="Clust (strict)"("Visible"=FALSE) -> ()  [unwired: 2 in, 2 out]
                n127 = local write "Test Name"(u16 0) -> ()
              }
            }
            n128 = property on="Test Tree" class="Tree (strict)"("Active Item Row Number"=w248, "ActiveColNum"=w248, "CellBG"=w245, "Active Item Row Number"=-1 ("Active Item:Row Number"), "CellBG"=u32 5789784 ("Color Box")) -> ()  [unwired: 2 in, 2 out]
          }
          frame "Variables" {
            w260 = string[] ["CameraPublisher", "Usage", "DB"]  # Items to initially close
            n129 = First Call?() -> (First Call?: T/F=w261:bool)
            n130 = control-ref of="Tree"() -> (w262:refnum<vi>)
            n131 = Select(t=w260, s=w261, f=string[] []) -> (s? t:f=w258:string[])
            n132 = call <vilib>:"NT Read and Format Entries as Tree.vi"("Tags to  Close"=w258, "Tree Refnum"=w262) -> ()  [unwired: 8 in, 2 out]
          }
          frame "Commands" {
            w271 = u32 5789784 ("Color Box")
            w272 = T28 {"Row"=-1, "Column"=-2} ("Active Cell:Active Cell")
            w274 = T28 {"Row"=-2, "Column"=-2} ("Active Cell:Active Cell")
            n133 = Index Array(array=w275, index=w269) -> (element=w273:u32)
            n134 = Index Array(array=w270, index=w269) -> (element=w268:T27)
            n135 = Unbundle(w268) -> ("Operation"=w267:enum16{"Update", "Clear"})  [unwired: 1 out]
            n136 = local read "Command Selection"() -> (w266:i32)
            n137 = property on="Command Selection" class="MCListbox (strict)"("ActiveCell"=w274, "CellBG"=w273, "ActiveCell"=w272, "CellBG"=w271) -> ()  [unwired: 2 in, 2 out]
            n138 = call <vilib>:"WPI_DashboardUpdate RPC Info.vi"("Operation"=w267) -> ("update"=w265:bool, "commands"=w264:string[][])  [unwired: 9 in]
            n139 = property on="Command Selection" class="MCListbox (strict)"("ItemNames"=w264) -> ()  [unwired: 2 in, 2 out]
            n140 = property on="Command Params" class="Tbl (strict)"("Active Cell"=w274, "Cell BG Color"=w273, "Active Cell"=w272, "Cell BG Color"=w271) -> ()  [unwired: 2 in, 2 out]
            n141 = call <vilib>:"WPI_DashboardUpdate Command Params.vi"("Update"=w265, "NewVal"=w266, "Commands"=w264, "Param Tbl"=w263) -> ()  [unwired: 7 in, 1 out]
          }
        }
        n142 = call <vilib>:"Connextion Info.vi"() -> ("Connected"=→"NT Connection":bool)  [unwired: 10 in, 1 out]
      }
      event "Test Tree": Value Change {
        # "Show appropriate\ncontrols"
        n143 = event-data() -> ("CtlRef"=w280:refnum<vi>, "NewVal"=w278:string)  [unwired: 1 in]
        n144 = call <vilib>:"WPI_UtilitiesGetTreeIOName.vi"("NewVal"=w278, "TreeControl in"=w280) -> ("I/O Name"=w281:string)  [unwired: 9 in]
        n145 = case shown="\"Camera\"" w281 {
          selector: w281 -> [_ w288 _ w310 w319 _]
          tunnel: w278 -> [_ _ w307 w309 _ w326]
          tunnel: cluster{string[]}[] [{["640x480", "320x240", "160x120"]}, {["Auto", "Fixed indoor", "Fixed outdoor 1", "Fixed outdoor 2", "Fixed fluorescent 1", "Fixed fluorescent 2", "Hold current"]}, {["Auto", "Flicker-free 50 Hz", "Flicker-free 60 Hz", "Hold current"]}, {["None", "Prioritize frame rate", "Prioritize image quality"]}, {["Monochrome", "Color"]}] -> [_ _ _ _ _ w325]
          frame Default {
            w283 = FALSE ("Visible")
            w282 = FALSE ("Visible")
            n146 = property on="Motor" class="Clust (strict)"("Visible"=w282) -> ()  [unwired: 2 in, 2 out]
            n147 = property on="Test Ring" class="Ring (strict)"("Visible"=w282) -> ()  [unwired: 2 in, 2 out]
            n148 = property on="Rev/Fwd" class="Clust (strict)"("Visible"=w283) -> ()  [unwired: 2 in, 2 out]
            n149 = property on="On/Off" class="Bool (strict)"("Visible"=w283) -> ()  [unwired: 2 in, 2 out]
            n150 = property on="Test Slider" class="Slide (strict)"("Visible"=w283) -> ()  [unwired: 2 in, 2 out]
          }
          frame "Analog Out", "Motor", "PWM" {
            w289 = FALSE ("Visible")
            n151 = case shown="\"Analog Out\"" w288 {
              tunnel: [1.0 ("Value") -1.0 ("Value") 0.0 ("Value")] -> w287
              tunnel: [255.0 ("Value") 1.0 ("Value") 5.0 ("Value")] -> w286
              tunnel: [128.0 ("Value") 0.0 ("Value") 0.0 ("Value")] -> w285
              tunnel: [64.0 ("Value") 0.5 ("Value") 1.0 ("Value")] -> w284
              frame "PWM" {
              }
              frame "Motor", Default {
              }
              frame "Analog Out" {
              }
            }
            n152 = property on="Motor" class="Clust (strict)"("Visible"=TRUE) -> ()  [unwired: 2 in, 2 out]
            n153 = property on="Value" class="Slide (strict)"("Value"=w285, "Scale.Minimum"=w287, "Scale.Maximum"=w286, "Scale.Increment"=w284) -> ()  [unwired: 2 in, 2 out]
            n154 = property on="On/Off" class="Bool (strict)"("Visible"=w289) -> ()  [unwired: 2 in, 2 out]
            n155 = property on="Test Slider" class="Slide (strict)"("Visible"=w289) -> ()  [unwired: 2 in, 2 out]
            n156 = property on="Test Ring" class="Ring (strict)"("Visible"=w289) -> ()  [unwired: 2 in, 2 out]
            n157 = property on="Rev/Fwd" class="Clust (strict)"("Visible"=w289) -> ()  [unwired: 2 in, 2 out]
          }
          frame "Servo" {
            w305 = FALSE ("Visible")
            n158 = call <vilib>:"NT Read Number.vi"("Name"=w307) -> ("Numeric"=w306:dbl)  [unwired: 9 in, 1 out]
            n159 = property on="Test Slider" class="Slide (strict)"("Visible"=TRUE, "Scale.Maximum"=170.0 ("Scale.Range:Maximum")) -> ()  [unwired: 2 in, 2 out]
            n160 = local write "Test Slider"(w306) -> ()
            n161 = property on="Motor" class="Clust (strict)"("Visible"=w305) -> ()  [unwired: 2 in, 2 out]
            n162 = property on="Rev/Fwd" class="Clust (strict)"("Visible"=w305) -> ()  [unwired: 2 in, 2 out]
            n163 = property on="On/Off" class="Bool (strict)"("Visible"=w305) -> ()  [unwired: 2 in, 2 out]
            n164 = property on="Test Ring" class="Ring (strict)"("Visible"=w305) -> ()  [unwired: 2 in, 2 out]
          }
          frame "Relay", "Solenoid" {
            w308 = FALSE ("Visible")
            n165 = property on="Motor" class="Clust (strict)"("Visible"=w308) -> ()  [unwired: 2 in, 2 out]
            n166 = property on="Test Slider" class="Slide (strict)"("Visible"=w308) -> ()  [unwired: 2 in, 2 out]
            n167 = Search and Replace String(input string=w309, search string="/Value  **", replace string="/Direction") -> (result string=w315:string)  [unwired: 5 in, 3 out]
            n168 = property on="Test Ring" class="Ring (strict)"("Visible"=w308) -> ()  [unwired: 2 in, 2 out]
            n169 = call <vilib>:"NT Read String.vi"("Name"=w315) -> ("String"=w313:string)  [unwired: 9 in, 1 out]
            n170 = Equal?(x="Both directions", y=w313) -> (x = y?=w311:bool)
            n171 = Not(x=w311) -> (.not. x?=w312:bool)
            n172 = property on="Rev/Fwd" class="Clust (strict)"("Visible"=w311) -> ()  [unwired: 2 in, 2 out]
            n173 = property on="On/Off" class="Bool (strict)"("Visible"=w312, "Caption.Text"=w310) -> ()  [unwired: 2 in, 2 out]
          }
          frame "Compressor", "Digital Out" {
            w318 = FALSE ("Visible")
            # "Get direction and finish"
            n174 = property on="Motor" class="Clust (strict)"("Visible"=w318) -> ()  [unwired: 2 in, 2 out]
            n175 = property on="Test Slider" class="Slide (strict)"("Visible"=w318) -> ()  [unwired: 2 in, 2 out]
            n176 = property on="Test Ring" class="Ring (strict)"("Visible"=w318) -> ()  [unwired: 2 in, 2 out]
            n177 = property on="On/Off" class="Bool (strict)"("Visible"=TRUE, "Caption.Text"=w319) -> ()  [unwired: 2 in, 2 out]
            n178 = property on="Rev/Fwd" class="Clust (strict)"("Visible"=FALSE) -> ()  [unwired: 2 in, 2 out]
          }
          frame "Camera" {
            n179 = call <vilib>:"Get Last Path Segment.vi"("String in"=w326) -> ("String out"=w327:string)  [unwired: 10 in]
            n180 = property on="On/Off" class="Bool (strict)"("Visible"=FALSE) -> ()  [unwired: 2 in, 2 out]
            n181 = property on="Motor" class="Clust (strict)"("Visible"=FALSE) -> ()  [unwired: 2 in, 2 out]
            n182 = property on="Rev/Fwd" class="Clust (strict)"("Visible"=FALSE) -> ()  [unwired: 2 in, 2 out]
            n183 = case shown="\"White Balance  **\"" w327 {
              tunnel: w326 -> [w333 w342 w351 w360 w369 _ w375]
              tunnel: w325 -> [w331 w339 w348 w357 w366 _ _]
              frame "Size  **" {
                n184 = Index Array(array=w331) -> (element=w330:cluster{string[]})  [unwired: 1 in]
                n185 = call <vilib>:"NT Read String.vi"("Name"=w333) -> ("String"=w332:string)  [unwired: 9 in, 1 out]
                n186 = Unbundle(w330) -> (w328:string[])
                n187 = Match First String(2:w328, 3:w332) -> (0:w329:i32)  [unwired: 1 out]
                n188 = property on="Test Ring" class="Ring (strict)"("Value"=w329, "Strings []"=w328) -> ()  [unwired: 2 in, 2 out]
                n189 = property on="Test Ring" class="Ring (strict)"("Visible"=TRUE) -> ()  [unwired: 2 in, 2 out]
                n190 = property on="Test Slider" class="Slide (strict)"("Visible"=FALSE) -> ()  [unwired: 2 in, 2 out]
              }
              frame "White Balance  **" {
                n191 = Index Array(array=w339, index=1) -> (element=w340:cluster{string[]})
                n192 = call <vilib>:"NT Read String.vi"("Name"=w342) -> ("String"=w341:string)  [unwired: 9 in, 1 out]
                n193 = Unbundle(w340) -> (w337:string[])
                n194 = Match First String(2:w337, 3:w341) -> (0:w336:i32)  [unwired: 1 out]
                n195 = property on="Test Ring" class="Ring (strict)"("Value"=w336, "Strings []"=w337) -> ()  [unwired: 2 in, 2 out]
                n196 = property on="Test Ring" class="Ring (strict)"("Visible"=TRUE) -> ()  [unwired: 2 in, 2 out]
                n197 = property on="Test Slider" class="Slide (strict)"("Visible"=FALSE) -> ()  [unwired: 2 in, 2 out]
              }
              frame "Exposure  **" {
                n198 = Index Array(array=w348, index=2) -> (element=w349:cluster{string[]})
                n199 = call <vilib>:"NT Read String.vi"("Name"=w351) -> ("String"=w350:string)  [unwired: 9 in, 1 out]
                n200 = Unbundle(w349) -> (w345:string[])
                n201 = Match First String(2:w345, 3:w350) -> (0:w346:i32)  [unwired: 1 out]
                n202 = property on="Test Ring" class="Ring (strict)"("Value"=w346, "Strings []"=w345) -> ()  [unwired: 2 in, 2 out]
                n203 = property on="Test Ring" class="Ring (strict)"("Visible"=TRUE) -> ()  [unwired: 2 in, 2 out]
                n204 = property on="Test Slider" class="Slide (strict)"("Visible"=FALSE) -> ()  [unwired: 2 in, 2 out]
              }
              frame "Exposure Priority  **" {
                n205 = Index Array(array=w357, index=3) -> (element=w358:cluster{string[]})
                n206 = call <vilib>:"NT Read String.vi"("Name"=w360) -> ("String"=w359:string)  [unwired: 9 in, 1 out]
                n207 = Unbundle(w358) -> (w354:string[])
                n208 = Match First String(2:w354, 3:w359) -> (0:w355:i32)  [unwired: 1 out]
                n209 = property on="Test Ring" class="Ring (strict)"("Value"=w355, "Strings []"=w354) -> ()  [unwired: 2 in, 2 out]
                n210 = property on="Test Ring" class="Ring (strict)"("Visible"=TRUE) -> ()  [unwired: 2 in, 2 out]
                n211 = property on="Test Slider" class="Slide (strict)"("Visible"=FALSE) -> ()  [unwired: 2 in, 2 out]
              }
              frame "Color Enable  **" {
                n212 = Index Array(array=w366, index=4) -> (element=w367:cluster{string[]})
                n213 = call <vilib>:"NT Read String.vi"("Name"=w369) -> ("String"=w368:string)  [unwired: 9 in, 1 out]
                n214 = Unbundle(w367) -> (w363:string[])
                n215 = Match First String(2:w363, 3:w368) -> (0:w364:i32)  [unwired: 1 out]
                n216 = property on="Test Ring" class="Ring (strict)"("Value"=w364, "Strings []"=w363) -> ()  [unwired: 2 in, 2 out]
                n217 = property on="Test Ring" class="Ring (strict)"("Visible"=TRUE) -> ()  [unwired: 2 in, 2 out]
                n218 = property on="Test Slider" class="Slide (strict)"("Visible"=FALSE) -> ()  [unwired: 2 in, 2 out]
              }
              frame Default {
                n219 = property on="Test Ring" class="Ring (strict)"("Visible"=FALSE) -> ()  [unwired: 2 in, 2 out]
                n220 = property on="Test Slider" class="Slide (strict)"("Visible"=FALSE) -> ()  [unwired: 2 in, 2 out]
              }
              frame "Brightness  **", "Color Level  **", "Compression  **", "FPS  **", "Sharpness  **" {
                n221 = call <vilib>:"NT Read Number.vi"("Name"=w375) -> ("Numeric"=w374:dbl)  [unwired: 9 in, 1 out]
                n222 = local write "Test Slider"(w374) -> ()
                n223 = property on="Test Slider" class="Slide (strict)"("Visible"=TRUE, "Scale.Maximum"=100.0 ("Scale.Range:Maximum")) -> ()  [unwired: 2 in, 2 out]
                n224 = property on="Test Ring" class="Ring (strict)"("Visible"=FALSE) -> ()  [unwired: 2 in, 2 out]
              }
            }
          }
        }
        n225 = property on="Progress" class="Clust (strict)"("Visible"=FALSE) -> ()  [unwired: 2 in, 2 out]
      }
      event "Test Name": Mouse Enter {
        # "Populate the ring with the list of tests"
        n226 = event-data() -> ()  [unwired: 1 in, 1 out]
        n227 = call <vilib>:"NT Read String Array.vi"("Name"="TestMode/TestList") -> ("String Array"=w383:string[])  [unwired: 9 in, 1 out]
        n228 = Build Array (concatenate)("Select the test to run...", w383) -> (w382:string[])
        n229 = property on="Test Name" class="Ring (strict)"("Strings []"=w382) -> ()  [unwired: 2 in, 2 out]
      }
      event "Test Name": Value Change {
        w385 = FALSE ("Visible")
        # "Tell the robot the test name to run"
        n230 = event-data() -> ("NewVal"=w389:u16)  [unwired: 1 in]
        n231 = property on="Test Name" class="Ring (strict)"() -> ("Strings []"=w390:string[])  [unwired: 2 in, 2 out]
        n232 = local write "Progress"(T9 {"Test Progress"=0, "Test Progress Text"=""} ("Progress")) -> ()
        n233 = Index Array(array=w390, index=w389) -> (element=w388:string)
        n234 = call <vilib>:"NT Write String.vi"("String"=w388, "Name"="TestMode/TestName") -> ()  [unwired: 9 in, 1 out]
        n235 = property on="Progress" class="Clust (strict)"("Visible"=TRUE) -> ()  [unwired: 2 in, 2 out]
        n236 = property on="Motor" class="Clust (strict)"("Visible"=w385) -> ()  [unwired: 2 in, 2 out]
        n237 = property on="Test Slider" class="Slide (strict)"("Visible"=w385) -> ()  [unwired: 2 in, 2 out]
        n238 = property on="On/Off" class="Bool (strict)"("Visible"=w385) -> ()  [unwired: 2 in, 2 out]
        n239 = property on="Rev/Fwd" class="Clust (strict)"("Visible"=w385) -> ()  [unwired: 2 in, 2 out]
        n240 = property on="Test Ring" class="Ring (strict)"("Visible"=w385) -> ()  [unwired: 2 in, 2 out]
      }
      event "Select Auto": Mouse Enter {
        # "Populate the combo box with the list of autonomous options"
        n241 = event-data() -> ()  [unwired: 1 in, 1 out]
        n242 = call <vilib>:"NT Read String Array.vi"("Name"="Auto List") -> ("String Array"=w392:string[])  [unwired: 9 in, 1 out]
        n243 = property on="Select Auto" class="CmbBox"("Strings[]"=w392) -> ()  [unwired: 2 in, 2 out]
      }
      event "Select Auto": Value Change {
        # "User modified the Auto Selection. Write to NT variable so robot knows."
        n244 = event-data() -> ("NewVal"=w395:string)  [unwired: 1 in]
        n245 = call <vilib>:"NT Write String.vi"("String"=w395, "Name"="Auto Selector") -> ()  [unwired: 9 in, 1 out]
      }
      event "Command Selection": Value Change {
        # "Get the params and show in table"
        n246 = event-data() -> ("NewVal"=w401:i32)  [unwired: 1 in]
        n247 = property on="Command Selection" class="MCListbox (strict)"() -> ("ItemNames"=w399:string[][])  [unwired: 2 in, 2 out]
        n248 = call <vilib>:"WPI_DashboardUpdate Command Params.vi"("NewVal"=w401, "Commands"=w399, "Param Tbl"=w400) -> ()  [unwired: 8 in, 1 out]
      }
      event "Execute Command": Value Change {
        # "Started one, Unique ID holds\nresponse"
        n249 = event-data() -> ()  [unwired: 1 in, 1 out]
        n250 = property on="Command Selection" class="MCListbox (strict)"() -> ("ItemNames"=w412:string[][])  [unwired: 2 in, 2 out]
        n251 = Index Array(array=w412, index (row)="Command Selection", index (col)=0) -> (element=w410:string)
        n252 = call <vilib>:"Invoke Commands.vi"("Command Params"="Command Params", "Function Name"=w410) -> ("Params"=w406:u8, "Started"=w405:bool)  [unwired: 7 in, 1 out]
        n253 = Array Subset(array="Command Params", length (row)=w406) -> (w407:string[][])  [unwired: 3 in]
        n254 = Select(t="Executing" ("Cmd Status"), s=w405, f="" ("Cmd Status")) -> (s? t:f=→"Cmd Status":string)
      }
      event "Command Selection": Double Click {
        n255 = event-data() -> ("Row"=w420:i32)  [unwired: 1 in]
        n256 = property on="Command Selection" class="MCListbox (strict)"() -> ("ItemNames"=w423:string[][])  [unwired: 2 in, 2 out]
        n257 = local read "Command Params"() -> (w419:string[][])
        n258 = Index Array(array=w423, index (row)=w420, index (col)=0) -> (element=w421:string)
        n259 = call <vilib>:"Invoke Commands.vi"("Command Params"=w419, "Function Name"=w421) -> ("Params"=w418:u8, "Started"=w413:bool)  [unwired: 7 in, 1 out]
        n260 = Array Subset(array=w419, length (row)=w418) -> (w417:string[][])  [unwired: 3 in]
        n261 = Select(t="Executing" ("Cmd Status"), s=w413, f="" ("Cmd Status")) -> (s? t:f=w414:string)
        n262 = local write "Cmd Status"(w414) -> ()
      }
      event "CheckList": Double Click {
        # "Shift clears all"
        # "Update symbols on the listbox"
        n263 = event-data() -> ("PlatMods.Shift"=w425:bool, "Row"=w427:i32)  [unwired: 1 in]
        n264 = case shown="True" w425 {
          tunnel: w427 -> [w431 _]
          tunnel: 1 -> [w430 _]
          frame False {
            n265 = property on="CheckList" class="LstBox (strict)"() -> ("Item Symbols"=w429:i32[])  [unwired: 2 in, 2 out]
            n266 = Replace Array Subset(array=w429, new element=w430, index=w431) -> (w428:i32[])
            n267 = property on="CheckList" class="LstBox (strict)"("Item Symbols"=w428) -> ()  [unwired: 2 in, 2 out]
          }
          frame True {
            w432 = 0 ("Top Row")
            n268 = property on="CheckList" class="LstBox (strict)"() -> ("Number of Rows"=w434:u32)  [unwired: 2 in, 2 out]
            n269 = Initialize Array(0, w434) -> (w433:i32[])
            n270 = property on="CheckList" class="LstBox (strict)"("Top Row"=w432, "Value"=w432, "Item Symbols"=w433) -> ()  [unwired: 2 in, 2 out]
          }
        }
      }
      event "CheckList": Key Down {
        # "Update symbols on the listbox\nLeft and right keys check and uncheck"
        n271 = event-data() -> ("VKey"=w438:T25)  [unwired: 1 in]
        n272 = case shown="\"Left\", \"Right\"" w438 {
          selector: w438 -> [w443 _]
          tunnel: eventvkey."Left" ("VKey") -> [w441 _]
          frame "Left", "Right" {
            n273 = Equal?(x=w441, y=w443) -> (x = y?=w442:bool)
            n274 = Select(t=0, s=w442, f=1) -> (s? t:f=w444:i32)
            n275 = property on="CheckList" class="LstBox (strict)"() -> ("Item Symbols"=w447:i32[])  [unwired: 2 in, 2 out]
            n276 = Replace Array Subset(array=w447, new element=w444, index="CheckList") -> (w446:i32[])
            n277 = property on="CheckList" class="LstBox (strict)"("Item Symbols"=w446) -> ()  [unwired: 2 in, 2 out]
          }
          frame Default {
          }
        }
      }
      event "Motor.Enable": Value Change {
        # "When the test mode otor enable helper is set, update that\ntree row item's value"
        n278 = event-data() -> ("NewVal"=w453:bool)  [unwired: 1 in]
        n279 = Unbundle("Motor") -> ("Value"=w452:dbl)  [unwired: 1 out]
        n280 = Select(t=w452, s=w453, f=0.0) -> (s? t:f=w450:dbl)
        n281 = call <vilib>:"NT Write Number.vi"("Numeric"=w450, "Name"=w449) -> ()  [unwired: 9 in, 1 out]
      }
      event "Test Slider": Value Change {
        # "When the test mode slider helper is set, update that\ntree row item's value"
        n282 = event-data() -> ("NewVal"=w456:dbl)  [unwired: 1 in]
        n283 = call <vilib>:"NT Write Number.vi"("Numeric"=w456, "Name"=w457) -> ()  [unwired: 9 in, 1 out]
      }
      event "On/Off": Value Change {
        # "When the test mode on/off helper value is set, update that\ntree row item's value"
        n284 = event-data() -> ("NewVal"=w461:bool)  [unwired: 1 in]
        n285 = Boolean To (0,1)(Boolean=w461) -> (0, 1=w460:i16)
        n286 = call <vilib>:"NT Write Number.vi"("Numeric"=w460, "Name"=w459) -> ()  [unwired: 9 in, 1 out]
      }
      event "Rev/Fwd": Value Change {
        # "When the test mode helper value for relays is set, update that\ntree row item's value"
        n287 = event-data() -> ("NewVal.Forward"=w469:bool, "NewVal.Reverse"=w468:bool)  [unwired: 1 in]
        n288 = Boolean To (0,1)(Boolean=w469) -> (0, 1=w465:i16)
        n289 = Boolean To (0,1)(Boolean=w468) -> (0, 1=w467:i16)
        n290 = Negate(x=w467) -> (-x=w466:i16)
        n291 = Add(x=w465, y=w466) -> (x+y=w464:i16)
        n292 = call <vilib>:"NT Write Number.vi"("Numeric"=w464, "Name"=w463) -> ()  [unwired: 9 in, 1 out]
      }
      event "Test Ring": Value Change {
        # "When a test mode helper value is selected from the ring,\nset the tree item's variable to the string value"
        n293 = event-data() -> ("NewVal"=w473:u16)  [unwired: 1 in]
        n294 = property on="Test Ring" class="Ring (strict)"() -> ("Strings []"=w474:string[])  [unwired: 2 in, 2 out]
        n295 = Index Array(array=w474, index=w473) -> (element=w472:string)
        n296 = call <vilib>:"NT Write String.vi"("String"=w472, "Name"=w471) -> ()  [unwired: 9 in, 1 out]
      }
      event "Rec Mode": Value Change {
        # "Update globals for recording mode and path to read log from.\nClear when logging and let NetworkTables set path for vision to\nuse."
        n297 = event-data() -> ("NewVal"=w485:enum32{"Stop", "Record", "Playback"})  [unwired: 1 in]
        n298 = global write "WPI_DashboardLogging Global.vi" "Logging Filename"(path "") -> ()
        n299 = global write "WPI_DashboardLogging Global.vi" "Recording"(w485) -> ()
        n300 = case shown="\"Playback\"" w485 {
          tunnel: w484 -> [_ w487 w496]
          tunnel: [_ _ w495] -> w482
          tunnel: [_ _ w494] -> _
          tunnel: w480 -> [_ _ w492]
          tunnel: cluster{i32, i32} {-250, 170} -> [_ _ w491]
          tunnel: [_ _ T26 {"Image Size"=TRUE, "Image Type"=TRUE, "Pixel Value"=TRUE, "ROI Information"=TRUE, "Zoom Factor"=FALSE} ("Image Information Shown:All Elements")] -> w475
          tunnel: [_ _ TRUE ("Zoom Factor")] -> w476
          tunnel: w478 -> [_ _ w488]
          frame Default {
          }
          frame "Stop", "Record" {
            # "Place Window too"
            n301 = invoke class="VI" method="FP.Close"(reference=w487) -> (reference out=w486:refnum<vi>)  [unwired: 2 in, 2 out]
            n302 = invoke class="VI" method="Abort VI"(reference=w486) -> ()  [unwired: 2 in, 3 out]
          }
          frame "Playback" {
            n303 = call "Open Playback Panel.vi"("Offset"=w491, "DB VI Ref"=w492, "Playback in"=w496) -> ("Playback out"=w493:refnum<vi>)  [unwired: 8 in]
            n304 = register-events(w493, w488) -> (reference out=w495:refnum<event-registration>, error out=w494:errorcluster)  [unwired: 2 in]
          }
        }
        n305 = property on="Camera Image Right" class="ImageControl"("Image Information Shown"=w475, "Image Information Visible"=w476) -> ()  [unwired: 2 in, 2 out]
        n306 = property on="Camera Image" class="ImageControl"("Image Information Shown"=w475, "Image Information Visible"=w476) -> ()  [unwired: 2 in, 2 out]
        n307 = call <vilib>:"WPI_DashboardNT Log FieldName Cache.vi"("Operation"=enum16{"Lookup/Add", "Index", "Clear"}."Clear") -> ()  [unwired: 8 in, 3 out]
      }
      event Panel Close {
        w498 = enum32{"Stop", "Record", "Playback"}."Stop" ("Rec Mode")
        # "Playback window has been closed, abort"
        n308 = event-data() -> ()  [unwired: 1 in, 4 out]
        n309 = local write "Rec Mode"(w498) -> ()
        n310 = global write "WPI_DashboardLogging Global.vi" "Recording"(w498) -> ()
      }
      event Panel Close {
        # "Abort playback window and ourself"
        n311 = event-data() -> ()  [unwired: 1 in, 4 out]
        n312 = invoke class="VI" method="FP.Close"(reference=w502) -> (reference out=w501:refnum<vi>)  [unwired: 2 in, 2 out]
        n313 = invoke class="VI" method="Abort VI"(reference=w501) -> (error out=w500:errorcluster)  [unwired: 2 in, 2 out]
        n314 = invoke class="VI" method="Abort VI"(error in=w500) -> ()  [unwired: 2 in, 3 out]
      }
      event User Event {
        n315 = event-data() -> ("IDs"=w509:cluster{"RPC field ID":u16, "Unique ID":u16}, "String"=w508:string)  [unwired: 1 in]
        n316 = Bundle("IDs"=w509, "String"=w508) -> (w507:T13)  [unwired: 1 in]
        n317 = call <vilib>:"Retrieve RPC Response.vi"("RPC Response"=w507) -> ("Output"=w505:string[][])  [unwired: 10 in]
        n318 = Build Array (concatenate)(w503, w505) -> (w504:string[][])
        n319 = local write "Command Params"(w504) -> ()
        n320 = local write "Cmd Status"("" ("Cmd Status")) -> ()
      }
      event "Tree": Double Click {
        n321 = event-data() -> ("PlatMods"=w515:T29, "Tag"=w512:string)  [unwired: 1 in]
        n322 = Unbundle(w515) -> ("Shift"=w514:bool)  [unwired: 4 out]
        n323 = String Subset(string=w512, length (rest)=1 ("length (rest)")) -> (substring=w511:string)  [unwired: 1 in]
        n324 = Not(x=w514) -> (.not. x?=w513:bool)
        n325 = case shown="\"/\"" w511 {
          tunnel: w512 -> [_ w518]
          tunnel: w513 -> [_ w517]
          frame Default {
          }
          frame "/" {
            n326 = call <vilib>:"NT Update Persistence.vi"("Persistence"=w517, "Name"=w518) -> ()  [unwired: 9 in, 1 out]
          }
        }
      }
    }
  }
  n327 = while {
    tunnel: w65 -> [w520]
    i -> [w523]
    stop <- FALSE stop-if-true
    n328 = Wait (ms)(milliseconds to wait=u32 100) -> ()  [unwired: 1 out]
    n329 = case shown="\"Playback\"" "Rec Mode" {
      tunnel: w523 -> [_ _ w538]
      tunnel: [u32 2829099 ("Base Color") u32 11141120 ("Target Color") w527] -> w519
      frame "Stop", Default {
        # "Reset the color, extra updates don't cost much"
      }
      frame "Record" {
      }
      frame "Playback" {
        # "Playback"
        n330 = Quotient & Remainder(x=w538, y=u32 50 ("milliseconds to wait")) -> (x-y*floor(x/y)=w534:u32)  [unwired: 1 out]
        n331 = Divide(x=w534, y=u32 50 ("milliseconds to wait")) -> (x/y=w531:dbl)
        n332 = Multiply(x=6.283185307179586, y=w531) -> (x*y=w536:dbl)
        n333 = Sine(x=w536) -> (sin(x)=w535:dbl)
        n334 = Absolute Value(x=w535) -> (abs(x)=w528:dbl)
        n335 = call "Interpolate RGB Color.vi"("Proportion"=w528, "Target Color"=u32 30976, "Base Color"=u32 2829099) -> ("Result Color"=w527:u32)  [unwired: 8 in]
      }
    }
    n336 = property class="Pane"(reference=w520, "PaneColor"=w519) -> ()  [unwired: 1 in, 2 out]
  }
  n337 = local write "Dashboard Tab"(T2."Drive" ("Dashboard Tab")) -> ()
  n338 = property on="On/Off" class="Bool (strict)"("Visible"=w36) -> ()  [unwired: 2 in, 2 out]
  n339 = property on="Motor" class="Clust (strict)"("Visible"=w36) -> ()  [unwired: 2 in, 2 out]
  n340 = property on="Progress" class="Clust (strict)"("Visible"=w36) -> ()  [unwired: 2 in, 2 out]
  n341 = property on="Test Ring" class="Ring (strict)"("Visible"=w36) -> ()  [unwired: 2 in, 2 out]
  n342 = property on="Rev/Fwd" class="Clust (strict)"("Visible"=w36) -> ()  [unwired: 2 in, 2 out]
  n343 = local write "Command Selection"(u16 0 ("milliseconds to wait")) -> ()
  n344 = while {
    tunnel: u16 1741 ("timeout ms (25000)") -> [w540]
    stop <- FALSE stop-if-true
    n345 = TCP Create Listener(10:w540) -> (0:w539:errorcluster, 3:w541:refnum<k5>)  [unwired: 4 in, 1 out]
    n346 = case shown="No Error" w539 {
      selector: w539 -> [w543 _]
      tunnel: w541 -> [w544 _]
      frame No Error {
        n347 = while {
          tunnel: w544 -> [w547]
          tunnel: w543 -> [w546]
          stop <- FALSE stop-if-true
          n348 = TCP Wait On Listener(8:w546, 11:w547) -> (0:w548:errorcluster, 4:w549:refnum<k5>)  [unwired: 2 in, 3 out]
          n349 = local write "TCP"(w549) -> ()
          n350 = case shown="No Error" w548 {
            frame No Error {
            }
            frame Error {
              n351 = Wait (ms)(milliseconds to wait=u32 1000) -> ()  [unwired: 1 out]
            }
          }
        }
      }
      frame Error {
        n352 = Wait (ms)(milliseconds to wait=u32 1000) -> ()  [unwired: 1 out]
      }
    }
  }
  n353 = local write "Command Params"(string[][] [] ("Command Params")) -> ()
  n354 = global write "WPI_DashboardLogging Global.vi" "Recording"(w59) -> ()
  n355 = local write "Rec Mode"(w59) -> ()
  n356 = call <vilib>:"NT Write String.vi"("String"="Select Auto", "Name"="Auto Selector") -> ()  [unwired: 9 in, 1 out]
